vi "DB_Action-GetModuleConfig.vi"(8 "error in":errorcluster, 11 "Name":string="A130") -> (0 "error out":errorcluster={"status"=TRUE, "code"=-2147467259, "source"="ADO Connection Open.vi->DB_Action.vi->DB_Action-GetModuleConfig.vi中的Exception occured in Microsoft JET Database Engine: 找不到文件 'E:\\FCT File Share\\29_WDML\\SO-20969 MSNG\\7_Code\\3_Software\\0_DB_Action\\WDML.mdb'。"}, 2 "Config":T1, 3 "Data":string[][](array[string]))   [LabVIEW 2015, in "Settings-Style.lvlib"]
uses:
  Settings-Style.lvlib
  1_Ctl/DB_UUT.ctl
  1_ctl/Ctl-Color.ctl
panel:
  # "Style Settings"
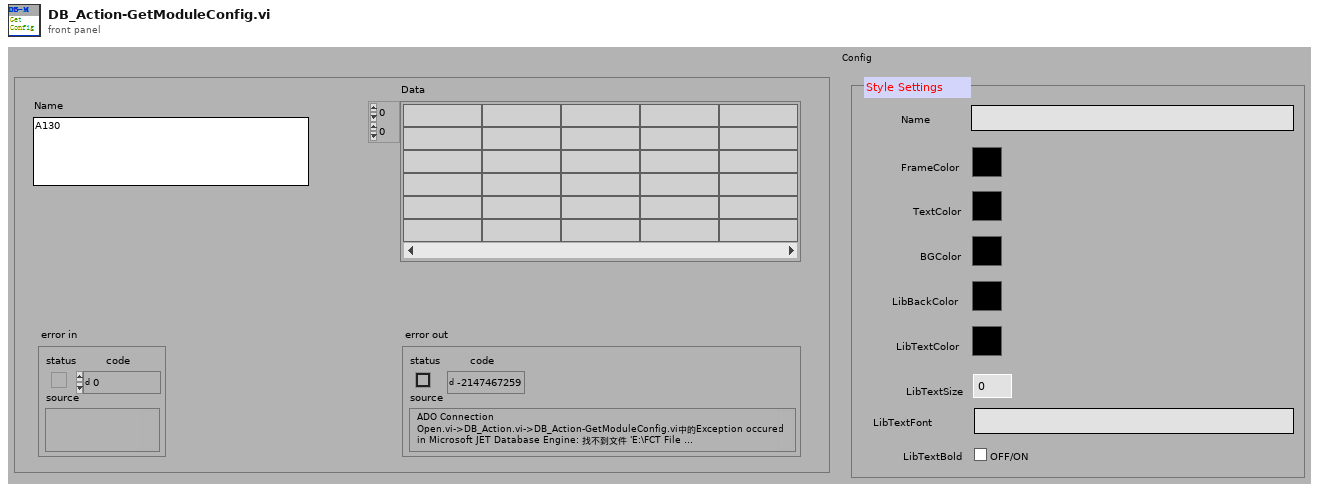
[diagram p1: front panel]
types:
  T1 = typedef "Settings-Style.lvlib/DB_UUT.ctl" = cluster{"Name":string, "FrameColor":T2, "TextColor":T2, "BGColor":T2, "LibBackColor":T2, "LibTextColor":T2, "LibTextSize":u32, "LibTextFont":string, "LibTextBold":bool}
  T2 = typedef "Ctl-Color.ctl" = u32
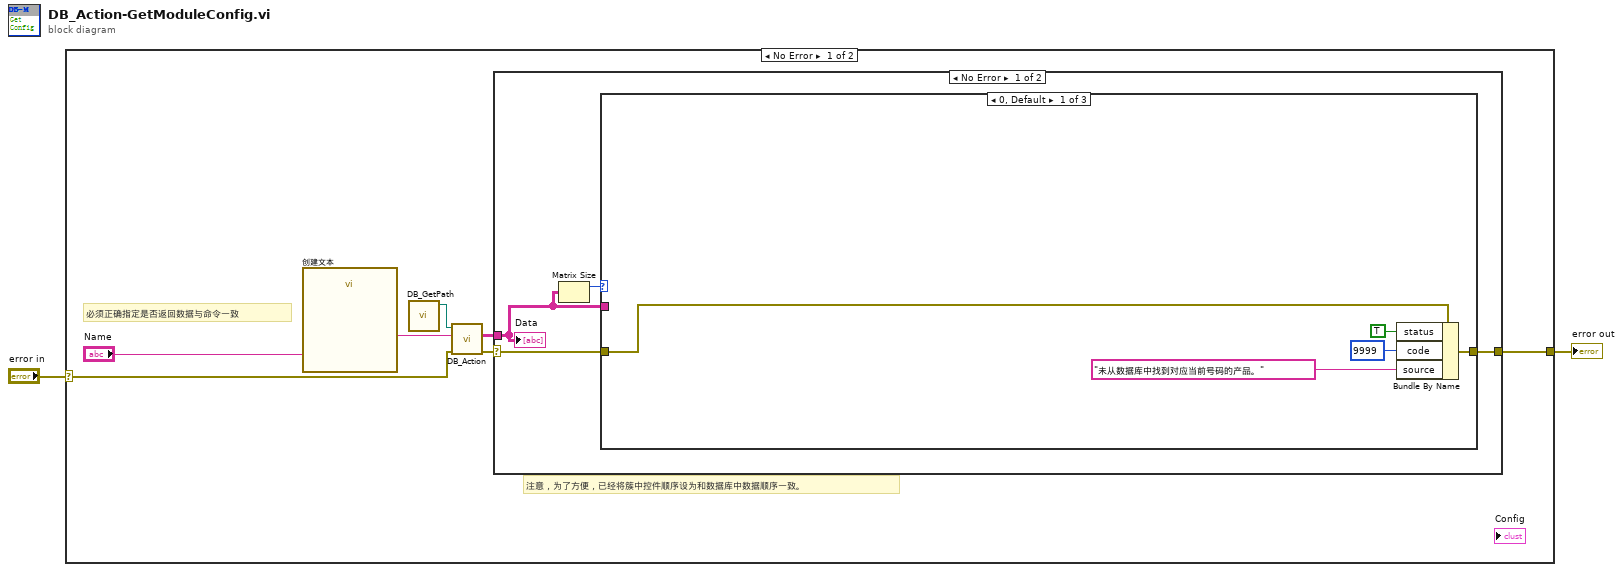
[diagram p0: block diagram]
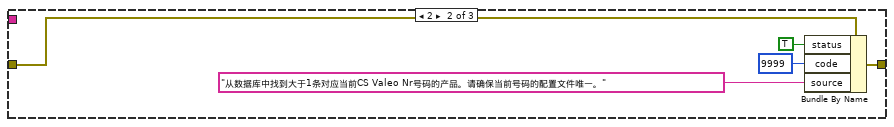
[diagram p2: hidden frame]
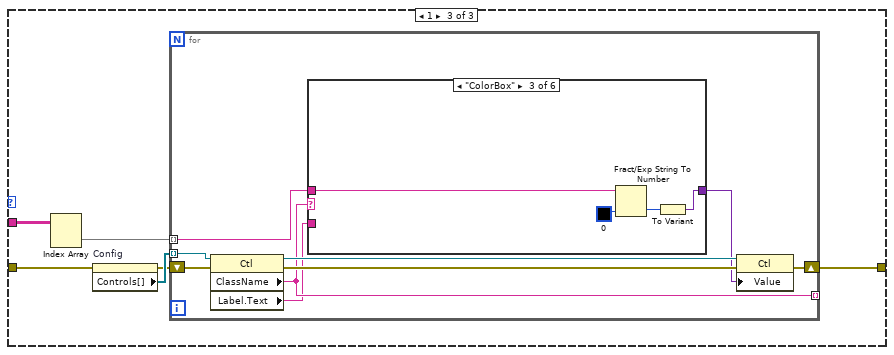
[diagram p3: hidden frame]
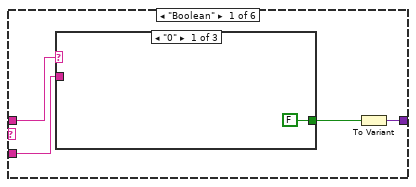
[diagram p4: hidden frame]
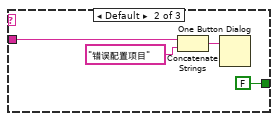
[diagram p5: hidden frame]
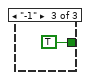
[diagram p6: hidden frame]
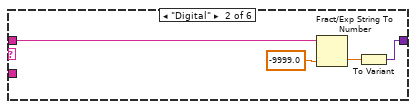
[diagram p7: hidden frame]
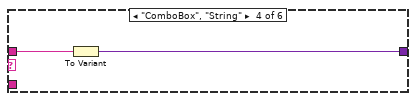
[diagram p8: hidden frame]
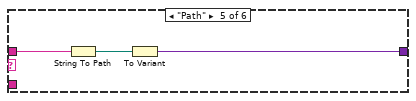
[diagram p9: hidden frame]
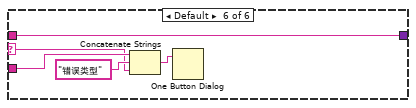
[diagram p10: hidden frame]
diagram:
  n1 = case shown="No Error" "error in" {
    selector: "error in" -> [w7 w68]
    tunnel: [w9 w68] -> w2
    frame No Error {
      # "注意，为了方便，已经将簇中控件顺序设为和数据库中数据顺序一致。"
      # "必须正确指定是否返回数据与命令一致"
      n2 = call "创建文本"("Name"="Name") -> ("Result"=w6:string)  [unwired: 13 in, 1 out]
      n3 = call "DB_GetPath.vi"() -> ("appended path"=w3:path)  [unwired: 11 in]
      n4 = call "DB_Action.vi"("error in"=w7, "Command Text"=w6, "路径"=w3) -> ("error out"=w5:errorcluster, "Data"=w4:string[][])  [unwired: 7 in]
      n5 = case shown="No Error" w5 {
        selector: w5 -> [w12 w67]
        tunnel: [w13 w67] -> w9
        tunnel: w4 -> [w11 _]
        frame No Error {
          n6 = Matrix Size(0:w11) -> (1:w10:i32)  [unwired: 1 out]
          n7 = case shown="0, Default" w10 {
            tunnel: w12 -> [w18 w20 w28]
            tunnel: [w17 w19 w26] -> w13
            tunnel: w11 -> [_ _ w24]
            frame 0, Default {
              n8 = Bundle By Name(cluster=w18, "status"=TRUE, "code"=9999, "source"="未从数据库中找到对应当前号码的产品。") -> (w17:errorcluster)
            }
            frame 2 {
              n9 = Bundle By Name(cluster=w20, "status"=TRUE, "code"=9999, "source"="从数据库中找到大于1条对应当前CS Valeo Nr号码的产品。请确保当前号码的配置文件唯一。") -> (w19:errorcluster)
            }
            frame 1 {
              n10 = Index Array(array=w24) -> (element=w25:string[])  [unwired: 2 in]
              n11 = property on="Config" class="Clust (strict)"(error in=w28) -> (error out=w27:errorcluster, "Controls[]"=w29:refnum<vi>[])  [unwired: 1 in, 1 out]
              n12 = for {
                tunnel: w29 -> [w38] mode=indexing
                tunnel: [w33] -> _ mode=indexing
                shift-right: [w35] -> w26
                shift-left: w27 -> [w34]
                tunnel: w25 -> [w32] mode=indexing
                n13 = property class="Ctl"(reference=w38, error in=w34) -> (reference out=w37:refnum<vi>, error out=w36:errorcluster, "ClassName"=w33:string, "Label.Text"=w30:string)
                n14 = case shown="\"ColorBox\"" w33 {
                  selector: w33 -> [_ _ _ _ _ w62]
                  tunnel: w32 -> [w42 w52 w56 w58 w61 w66]
                  tunnel: [w40 w49 w54 w57 w60 w66] -> w31
                  tunnel: w30 -> [w39 _ _ _ _ w65]
                  frame "Boolean" {
                    n15 = case shown="\"0\"" w42 {
                      tunnel: [FALSE FALSE TRUE] -> w41
                      tunnel: w39 -> [_ w46 _]
                      frame "0" {
                      }
                      frame Default {
                        n16 = Concatenate Strings(w46, "错误配置项目" ("消息")) -> (w44:string)
                        n17 = One Button Dialog(message=w44) -> ()  [unwired: 1 in, 1 out]
                      }
                      frame "-1" {
                      }
                    }
                    n18 = To Variant(anything=w41) -> (Variant=w40:variant)
                  }
                  frame "Digital" {
                    n19 = Fract/Exp String To Number(string=w52, default (0 dbl)=-9999.0 ("默认(0 DBL)")) -> (number=w50:dbl)  [unwired: 2 in, 1 out]
                    n20 = To Variant(anything=w50) -> (Variant=w49:variant)
                  }
                  frame "ColorBox" {
                    n21 = Fract/Exp String To Number(string=w56, default (0 dbl)=u32 0 ("Color Box")) -> (number=w55:u32)  [unwired: 2 in, 1 out]
                    n22 = To Variant(anything=w55) -> (Variant=w54:variant)
                  }
                  frame "ComboBox", "String" {
                    n23 = To Variant(anything=w58) -> (Variant=w57:variant)
                  }
                  frame "Path" {
                    n24 = String To Path(string=w61) -> (path=w59:path)
                    n25 = To Variant(anything=w59) -> (Variant=w60:variant)
                  }
                  frame Default {
                    n26 = Concatenate Strings(w65, "错误类型" ("消息"), w62) -> (w63:string)
                    n27 = One Button Dialog(message=w63) -> ()  [unwired: 1 in, 1 out]
                  }
                }
                n28 = property class="Ctl"(reference=w37, error in=w36, "Value"=w31) -> (error out=w35:errorcluster)  [unwired: 1 out]
              }
            }
          }
          "Data" <- w11
        }
        frame Error {
        }
      }
    }
    frame Error {
    }
  }
  "error out" <- w2
